vi "FGV_DOCK_controls_state.vi"(7 "options":T1, 8 "error_in":errorcluster, 11 "input":variant) -> (0 "error_out":errorcluster, 3 "output":variant)   [LabVIEW 2019]
uses:
  FGV_DOCK_controls_state.ctl
  FGV_DOCK_controls_state_refnums.ctl
  FGV_DOCK_controls_state_variables.ctl
  _misc/AULocalize/SubVIs/Get Localized Phrase Compact Interface 0D.vi
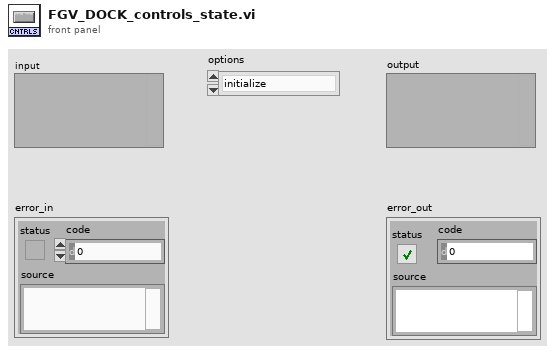
[diagram p1: front panel]
types:
  T1 = typedef "FGV_DOCK_controls_state.ctl" = enum16{"initialize", "login_event", "translation_event", "batch_event", "reload_event", "gear_event", "gear_saved_event", "gear_in_another_batch_event", "gear_in_current_batch_event", "NOK_ref_gear_event", "NOK_station_gear_event", "get_gear_loaded_status"}
  T2 = typedef "FGV_DOCK_controls_state_variables.ctl" = cluster{"access_level":i32, "batch_active?":bool, "gear_loaded?":bool}
  T3 = typedef "FGV_DOCK_controls_state_refnums.ctl" = cluster{"REFERENCE_selector":refnum<vi>, "BATCH_SIZE_selector":refnum<vi>, "DOCK_start_finish_batch":refnum<vi>, "gear_OK":refnum<vi>, "gear_NOK":refnum<vi>, "reload_part_number":refnum<vi>, "reload_batch_size":refnum<vi>, "menu_bar":refnum<k9>}
  T4 = enum8{"Enabled", "Disabled", "Disabled and Grayed Out"}
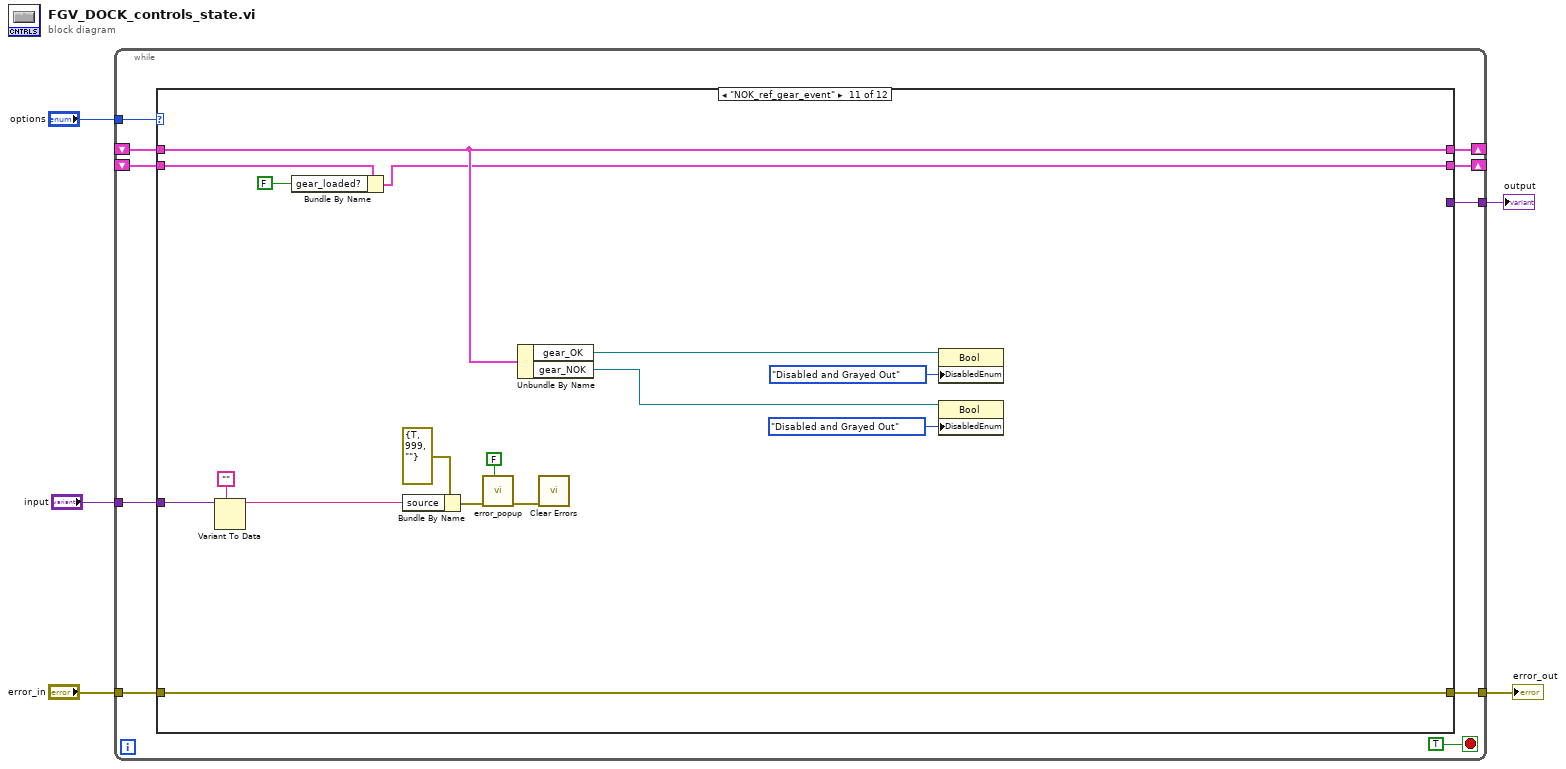
[diagram p0: block diagram]
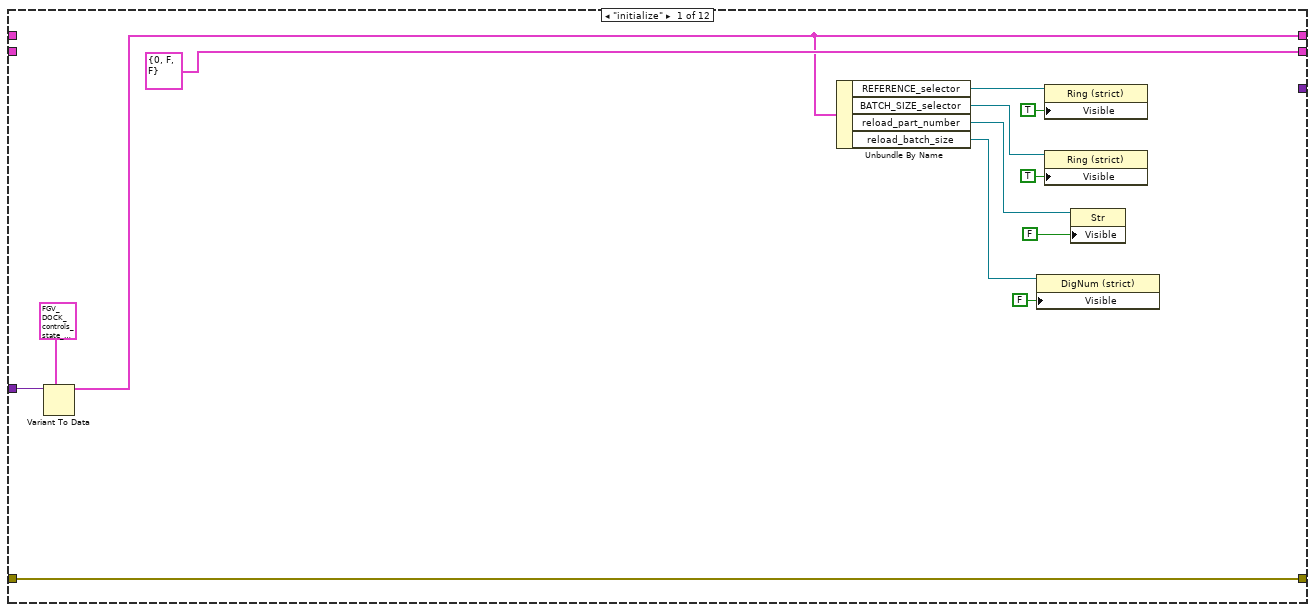
[diagram p2: hidden frame]
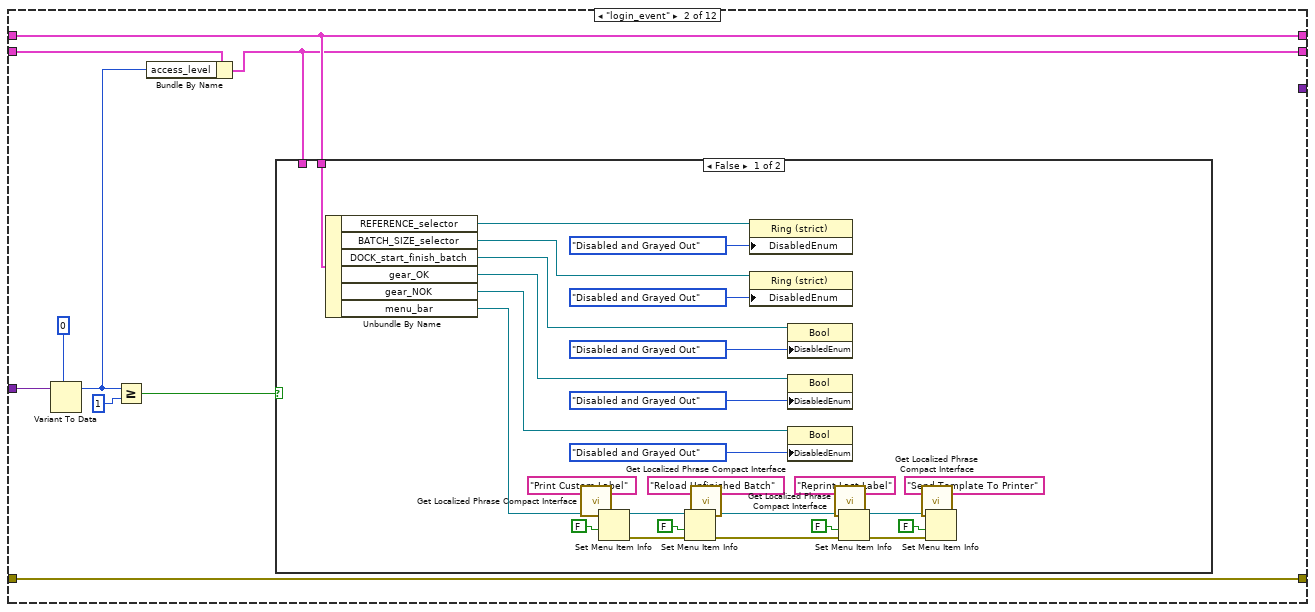
[diagram p3: hidden frame]
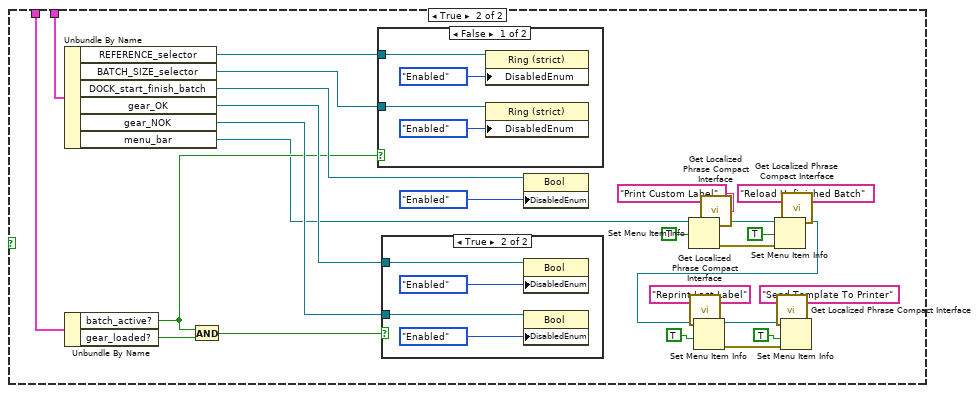
[diagram p4: hidden frame]
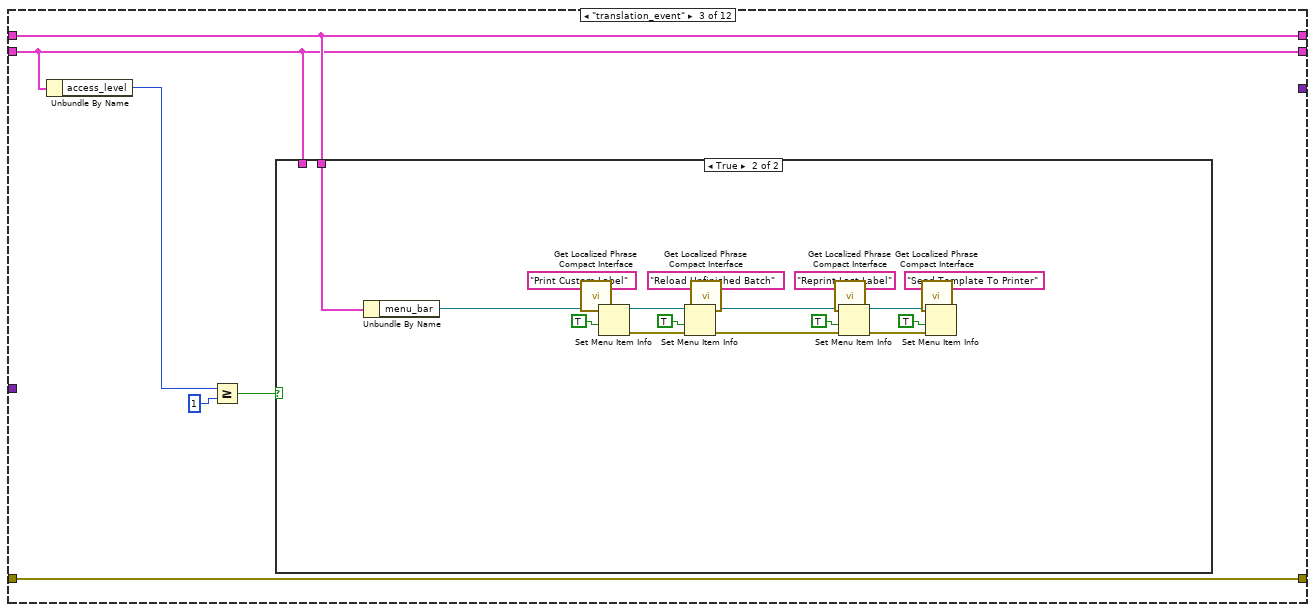
[diagram p7: hidden frame]
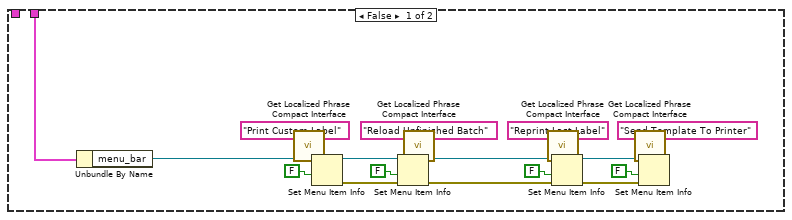
[diagram p8: hidden frame]
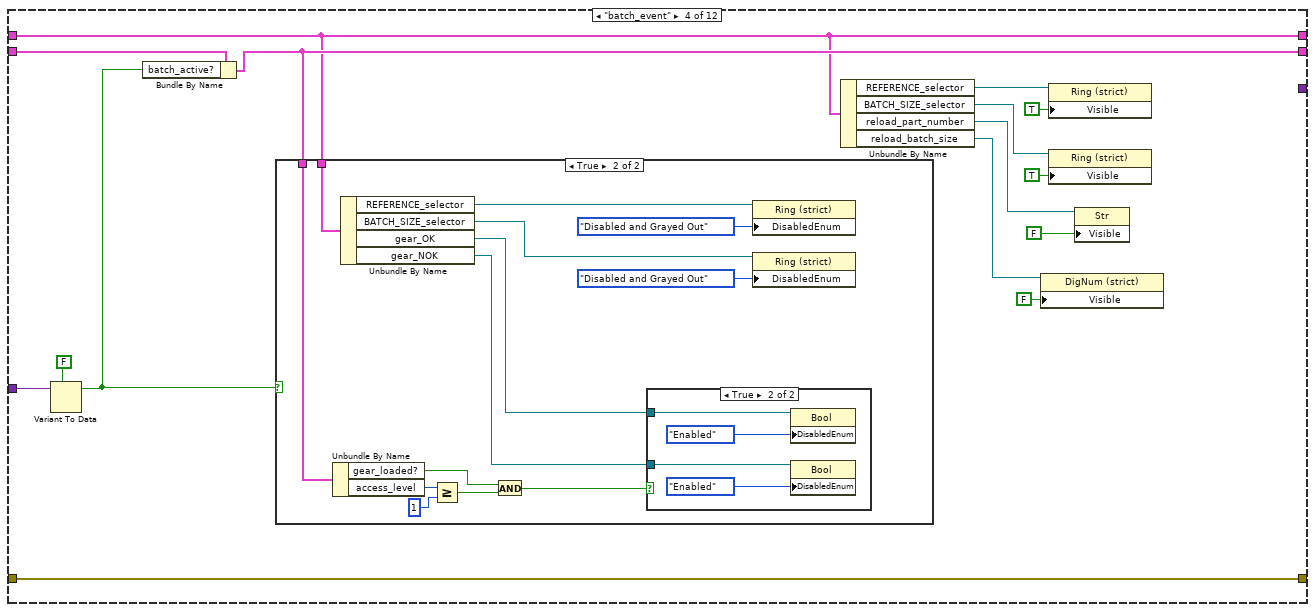
[diagram p9: hidden frame]
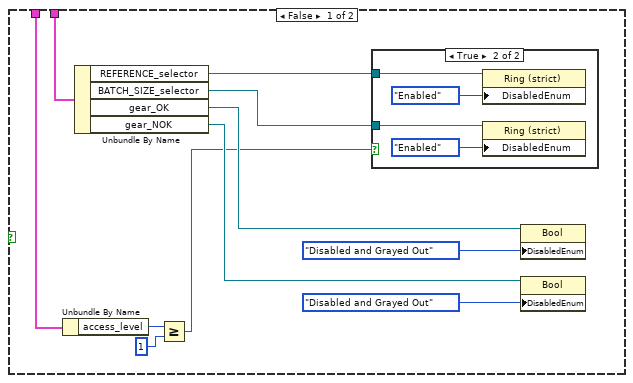
[diagram p10: hidden frame]
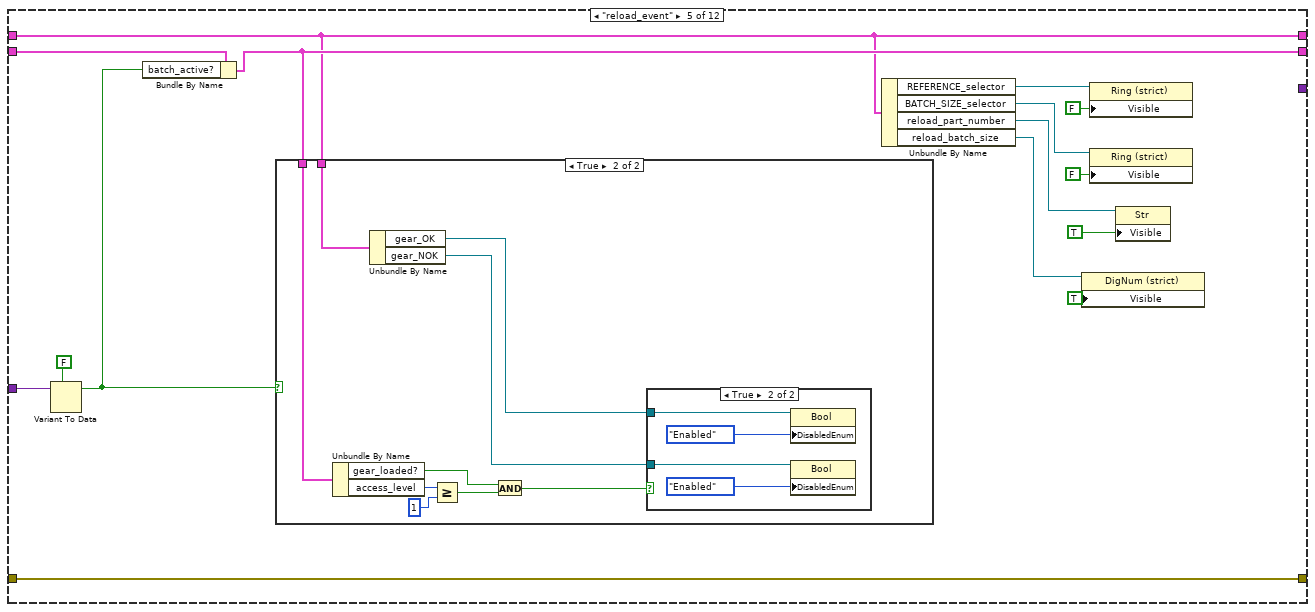
[diagram p13: hidden frame]
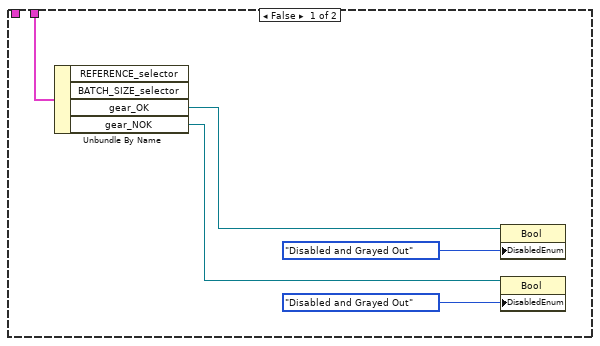
[diagram p14: hidden frame]
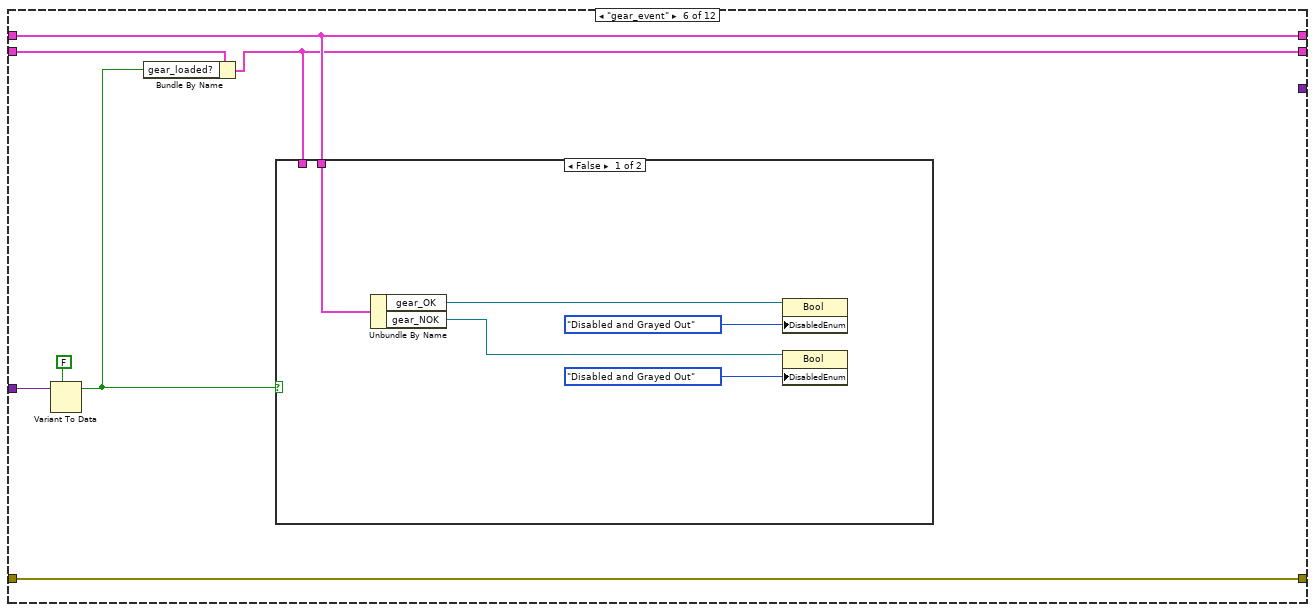
[diagram p16: hidden frame]
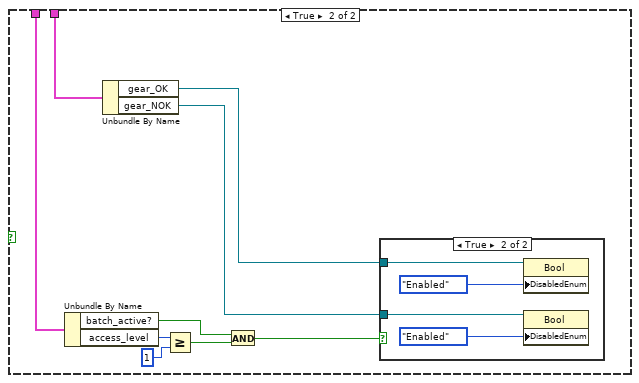
[diagram p17: hidden frame]
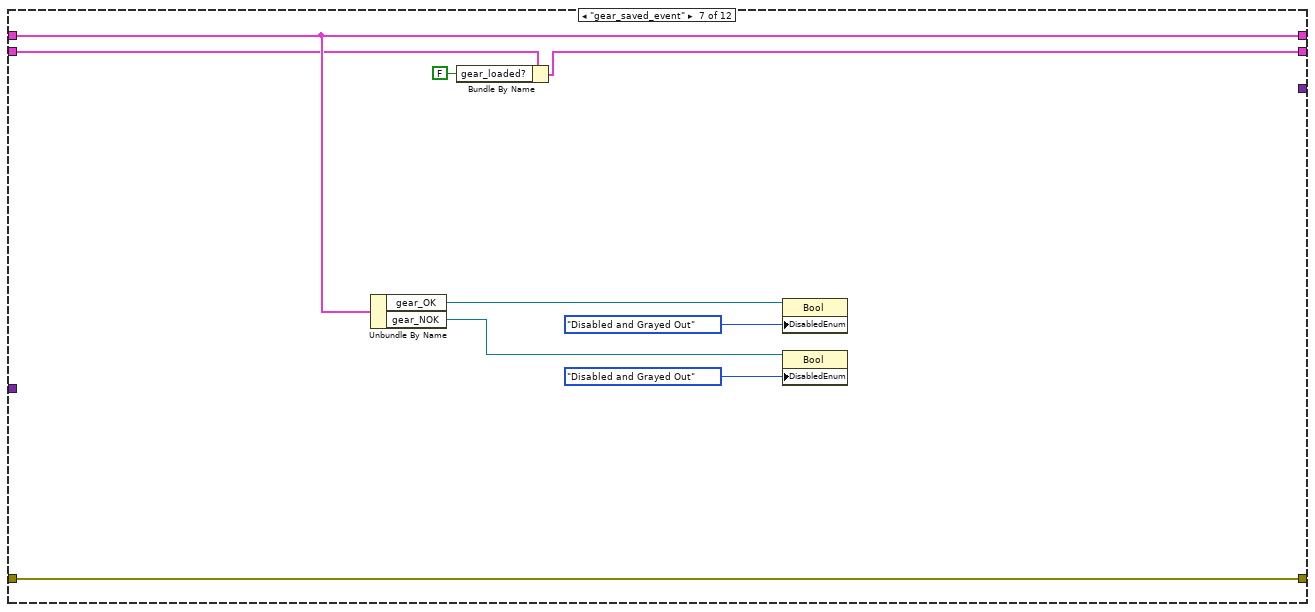
[diagram p19: hidden frame]
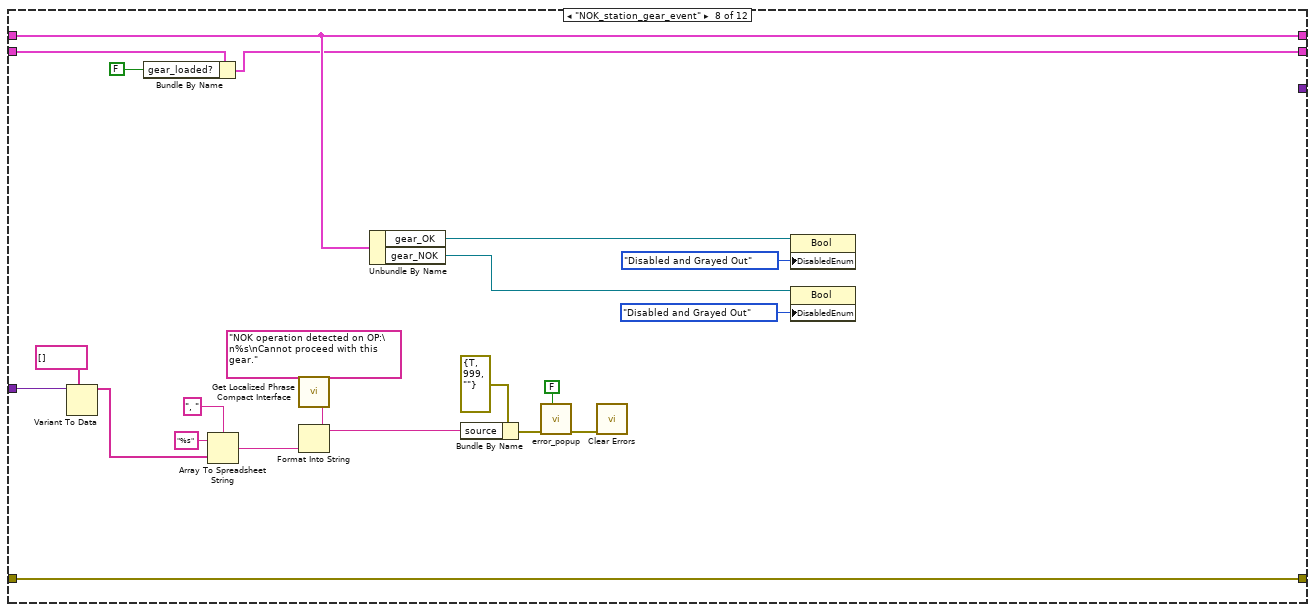
[diagram p20: hidden frame]
diagram:
  n1 = while {
    tunnel: "options" -> [w14]
    tunnel: [w13] -> w5
    tunnel: "error_in" -> [w12]
    tunnel: "input" -> [w11]
    shift-right: [w10] -> _
    shift-left: _ -> [w9]
    shift-right: [w8] -> _
    shift-left: _ -> [w7]
    tunnel: [w6] -> w1
    stop <- TRUE stop-if-true
    n2 = case shown="\"NOK_ref_gear_event\"" w14 {
      tunnel: [w28 w37 w110 w165 w212 w237 w264 w286 w298 w328 w344 w349] -> w13
      tunnel: w12 -> [w28 w37 w110 w165 w212 w237 w264 w286 w298 w328 w344 w349]
      tunnel: w11 -> [w27 w36 _ w164 w211 w236 _ w276 w293 _ w334 _]
      tunnel: [w16 w30 w107 w157 w198 w234 w263 w284 w297 w326 w342 w348] -> w10
      tunnel: w9 -> [_ w30 w107 w157 w198 w234 w263 w284 w297 w326 w342 w348]
      tunnel: [T2 {"access_level"=0, "batch_active?"=FALSE, "gear_loaded?"=FALSE} ("controls_state_variables") w29 w106 w162 w209 w233 w257 w283 w287 w325 w341 w347] -> w8
      tunnel: w7 -> [_ w32 w106 w163 w210 w235 w258 w285 w288 w327 w343 w347]
      tunnel: [_ _ _ _ _ _ _ _ _ _ _ w345] -> w6
      frame "initialize" {
        n3 = Variant To Data(type=T3 {"REFERENCE_selector"=refnum, "BATCH_SIZE_selector"=refnum, "DOCK_start_finish_batch"=refnum, "gear_OK"=refnum, "gear_NOK"=refnum, "reload_part_number"=refnum, "reload_batch_size"=refnum, "menu_bar"=refnum} ("control_refnums"), Variant=w27) -> (data=w16:T3)  [unwired: 1 in, 1 out]
        n4 = Unbundle By Name(w16) -> ("REFERENCE_selector"=w22:refnum<vi>, "BATCH_SIZE_selector"=w21:refnum<vi>, "reload_part_number"=w18:refnum<vi>, "reload_batch_size"=w17:refnum<vi>)
        n5 = property class="DigNum (strict)"(reference=w17, "Visible"=FALSE) -> ()  [unwired: 1 in, 2 out]
        n6 = property class="Ring (strict)"(reference=w22, "Visible"=TRUE) -> ()  [unwired: 1 in, 2 out]
        n7 = property class="Ring (strict)"(reference=w21, "Visible"=TRUE) -> ()  [unwired: 1 in, 2 out]
        n8 = property class="Str"(reference=w18, "Visible"=FALSE) -> ()  [unwired: 1 in, 2 out]
      }
      frame "login_event" {
        n9 = Variant To Data(type=0 ("y"), Variant=w36) -> (data=w31:i32)  [unwired: 1 in, 1 out]
        n10 = Greater Or Equal?(x=w31, y=1) -> (x >= y?=w33:bool)
        n11 = Bundle By Name(cluster=w32, "access_level"=w31) -> (w29:T2)
        n12 = case shown="False" w33 {
          tunnel: w30 -> [w66 w96]
          tunnel: w29 -> [_ w90]
          frame False {
            n13 = Unbundle By Name(w66) -> ("REFERENCE_selector"=w61:refnum<vi>, "BATCH_SIZE_selector"=w60:refnum<vi>, "DOCK_start_finish_batch"=w59:refnum<vi>, "gear_OK"=w58:refnum<vi>, "gear_NOK"=w57:refnum<vi>, "menu_bar"=w50:refnum<k9>)
            n14 = call-poly "Get Localized Phrase Compact Interface.vi"("Key"="Print Custom Label" ("item tag")) -> ("Translated Phrase"=w41:string)
            n15 = Set Menu Item Info(7:w41, 9:FALSE ("enabled"), 11:w50) -> (0:w52:errorcluster, 3:w51:refnum<k9>)  [unwired: 4 in]
            n16 = call-poly "Get Localized Phrase Compact Interface.vi"("Key"="Reload Unfinished Batch" ("item tag")) -> ("Translated Phrase"=w40:string)
            n17 = Set Menu Item Info(7:w40, 8:w52, 9:FALSE ("enabled"), 11:w51) -> (0:w45:errorcluster, 3:w44:refnum<k9>)  [unwired: 3 in]
            n18 = property class="Ring (strict)"(reference=w61, "DisabledEnum"=T4."Disabled and Grayed Out" ("Disabled")) -> ()  [unwired: 1 in, 2 out]
            n19 = property class="Ring (strict)"(reference=w60, "DisabledEnum"=T4."Disabled and Grayed Out" ("Disabled")) -> ()  [unwired: 1 in, 2 out]
            n20 = property class="Bool"(reference=w59, "DisabledEnum"=T4."Disabled and Grayed Out" ("Disabled")) -> ()  [unwired: 1 in, 2 out]
            n21 = property class="Bool"(reference=w58, "DisabledEnum"=T4."Disabled and Grayed Out" ("Disabled")) -> ()  [unwired: 1 in, 2 out]
            n22 = property class="Bool"(reference=w57, "DisabledEnum"=T4."Disabled and Grayed Out" ("Disabled")) -> ()  [unwired: 1 in, 2 out]
            n23 = call-poly "Get Localized Phrase Compact Interface.vi"("Key"="Reprint Last Label") -> ("Translated Phrase"=w39:string)
            n24 = Set Menu Item Info(7:w39, 8:w45, 9:FALSE ("enabled"), 11:w44) -> (0:w48:errorcluster, 3:w49:refnum<k9>)  [unwired: 3 in]
            n25 = call-poly "Get Localized Phrase Compact Interface.vi"("Key"="Send Template To Printer") -> ("Translated Phrase"=w38:string)
            n26 = Set Menu Item Info(7:w38, 8:w48, 9:FALSE ("enabled"), 11:w49) -> ()  [unwired: 3 in, 2 out]
          }
          frame True {
            n27 = Unbundle By Name(w96) -> ("REFERENCE_selector"=w95:refnum<vi>, "BATCH_SIZE_selector"=w94:refnum<vi>, "DOCK_start_finish_batch"=w93:refnum<vi>, "gear_OK"=w92:refnum<vi>, "gear_NOK"=w91:refnum<vi>, "menu_bar"=w79:refnum<k9>)
            n28 = Unbundle By Name(w90) -> ("batch_active?"=w88:bool, "gear_loaded?"=w87:bool)
            n29 = And(x=w88, y=w87) -> (x .and. y?=w86:bool)
            n30 = case shown="False" w88 {
              tunnel: w95 -> [w98 _]
              tunnel: w94 -> [w97 _]
              frame False {
                n31 = property class="Ring (strict)"(reference=w98, "DisabledEnum"=T4."Enabled" ("Disabled")) -> ()  [unwired: 1 in, 2 out]
                n32 = property class="Ring (strict)"(reference=w97, "DisabledEnum"=T4."Enabled" ("Disabled")) -> ()  [unwired: 1 in, 2 out]
              }
              frame True {
              }
            }
            n33 = case shown="True" w86 {
              tunnel: w92 -> [_ w102]
              tunnel: w91 -> [_ w101]
              frame False {
              }
              frame True {
                n34 = property class="Bool"(reference=w102, "DisabledEnum"=T4."Enabled" ("Disabled")) -> ()  [unwired: 1 in, 2 out]
                n35 = property class="Bool"(reference=w101, "DisabledEnum"=T4."Enabled" ("Disabled")) -> ()  [unwired: 1 in, 2 out]
              }
            }
            n36 = property class="Bool"(reference=w93, "DisabledEnum"=T4."Enabled" ("Disabled")) -> ()  [unwired: 1 in, 2 out]
            n37 = call-poly "Get Localized Phrase Compact Interface.vi"("Key"="Reprint Last Label") -> ("Translated Phrase"=w68:string)
            n38 = call-poly "Get Localized Phrase Compact Interface.vi"("Key"="Print Custom Label" ("item tag")) -> ("Translated Phrase"=w71:string)
            n39 = Set Menu Item Info(7:w71, 9:TRUE ("enabled"), 11:w79) -> (0:w85:errorcluster, 3:w84:refnum<k9>)  [unwired: 4 in]
            n40 = call-poly "Get Localized Phrase Compact Interface.vi"("Key"="Send Template To Printer") -> ("Translated Phrase"=w69:string)
            n41 = call-poly "Get Localized Phrase Compact Interface.vi"("Key"="Reload Unfinished Batch" ("item tag")) -> ("Translated Phrase"=w70:string)
            n42 = Set Menu Item Info(7:w70, 8:w85, 9:TRUE ("enabled"), 11:w84) -> (3:w72:refnum<k9>)  [unwired: 3 in, 1 out]
            n43 = Set Menu Item Info(7:w68, 9:TRUE ("enabled"), 11:w72) -> (0:w77:errorcluster, 3:w78:refnum<k9>)  [unwired: 4 in]
            n44 = Set Menu Item Info(7:w69, 8:w77, 9:TRUE ("enabled"), 11:w78) -> ()  [unwired: 3 in, 2 out]
          }
        }
      }
      frame "translation_event" {
        n45 = Unbundle By Name(w106) -> ("access_level"=w105:i32)
        n46 = Greater Or Equal?(x=w105, y=1) -> (x >= y?=w108:bool)
        n47 = case shown="True" w108 {
          tunnel: w107 -> [w130 w150]
          tunnel: w106 -> [_ _]
          frame False {
            n48 = Unbundle By Name(w130) -> ("menu_bar"=w123:refnum<k9>)
            n49 = call-poly "Get Localized Phrase Compact Interface.vi"("Key"="Print Custom Label" ("item tag")) -> ("Translated Phrase"=w114:string)
            n50 = Set Menu Item Info(7:w114, 9:FALSE ("enabled"), 11:w123) -> (0:w125:errorcluster, 3:w124:refnum<k9>)  [unwired: 4 in]
            n51 = call-poly "Get Localized Phrase Compact Interface.vi"("Key"="Reload Unfinished Batch" ("item tag")) -> ("Translated Phrase"=w113:string)
            n52 = Set Menu Item Info(7:w113, 8:w125, 9:FALSE ("enabled"), 11:w124) -> (0:w118:errorcluster, 3:w117:refnum<k9>)  [unwired: 3 in]
            n53 = call-poly "Get Localized Phrase Compact Interface.vi"("Key"="Reprint Last Label") -> ("Translated Phrase"=w112:string)
            n54 = Set Menu Item Info(7:w112, 8:w118, 9:FALSE ("enabled"), 11:w117) -> (0:w121:errorcluster, 3:w122:refnum<k9>)  [unwired: 3 in]
            n55 = call-poly "Get Localized Phrase Compact Interface.vi"("Key"="Send Template To Printer") -> ("Translated Phrase"=w111:string)
            n56 = Set Menu Item Info(7:w111, 8:w121, 9:FALSE ("enabled"), 11:w122) -> ()  [unwired: 3 in, 2 out]
          }
          frame True {
            n57 = Unbundle By Name(w150) -> ("menu_bar"=w143:refnum<k9>)
            n58 = call-poly "Get Localized Phrase Compact Interface.vi"("Key"="Print Custom Label" ("item tag")) -> ("Translated Phrase"=w134:string)
            n59 = Set Menu Item Info(7:w134, 9:TRUE ("enabled"), 11:w143) -> (0:w145:errorcluster, 3:w144:refnum<k9>)  [unwired: 4 in]
            n60 = call-poly "Get Localized Phrase Compact Interface.vi"("Key"="Reload Unfinished Batch" ("item tag")) -> ("Translated Phrase"=w133:string)
            n61 = Set Menu Item Info(7:w133, 8:w145, 9:TRUE ("enabled"), 11:w144) -> (0:w138:errorcluster, 3:w137:refnum<k9>)  [unwired: 3 in]
            n62 = call-poly "Get Localized Phrase Compact Interface.vi"("Key"="Reprint Last Label") -> ("Translated Phrase"=w132:string)
            n63 = Set Menu Item Info(7:w132, 8:w138, 9:TRUE ("enabled"), 11:w137) -> (0:w141:errorcluster, 3:w142:refnum<k9>)  [unwired: 3 in]
            n64 = call-poly "Get Localized Phrase Compact Interface.vi"("Key"="Send Template To Printer") -> ("Translated Phrase"=w131:string)
            n65 = Set Menu Item Info(7:w131, 8:w141, 9:TRUE ("enabled"), 11:w142) -> ()  [unwired: 3 in, 2 out]
          }
        }
      }
      frame "batch_event" {
        n66 = Variant To Data(type=FALSE, Variant=w164) -> (data=w160:bool)  [unwired: 1 in, 1 out]
        n67 = Bundle By Name(cluster=w163, "batch_active?"=w160) -> (w162:T2)
        n68 = case shown="True" w160 {
          tunnel: w157 -> [w176 w193]
          tunnel: w162 -> [w167 w188]
          frame False {
            n69 = Unbundle By Name(w167) -> ("access_level"=w168:i32)
            n70 = Unbundle By Name(w176) -> ("REFERENCE_selector"=w173:refnum<vi>, "BATCH_SIZE_selector"=w172:refnum<vi>, "gear_OK"=w171:refnum<vi>, "gear_NOK"=w170:refnum<vi>)
            n71 = Greater Or Equal?(x=w168, y=1) -> (x >= y?=w166:bool)
            n72 = case shown="True" w166 {
              tunnel: w173 -> [_ w178]
              tunnel: w172 -> [_ w177]
              frame False {
              }
              frame True {
                n73 = property class="Ring (strict)"(reference=w178, "DisabledEnum"=T4."Enabled" ("Disabled")) -> ()  [unwired: 1 in, 2 out]
                n74 = property class="Ring (strict)"(reference=w177, "DisabledEnum"=T4."Enabled" ("Disabled")) -> ()  [unwired: 1 in, 2 out]
              }
            }
            n75 = property class="Bool"(reference=w171, "DisabledEnum"=T4."Disabled and Grayed Out" ("Disabled")) -> ()  [unwired: 1 in, 2 out]
            n76 = property class="Bool"(reference=w170, "DisabledEnum"=T4."Disabled and Grayed Out" ("Disabled")) -> ()  [unwired: 1 in, 2 out]
          }
          frame True {
            n77 = Unbundle By Name(w188) -> ("gear_loaded?"=w182:bool, "access_level"=w184:i32)
            n78 = Unbundle By Name(w193) -> ("REFERENCE_selector"=w192:refnum<vi>, "BATCH_SIZE_selector"=w191:refnum<vi>, "gear_OK"=w190:refnum<vi>, "gear_NOK"=w189:refnum<vi>)
            n79 = Greater Or Equal?(x=w184, y=1) -> (x >= y?=w183:bool)
            n80 = And(x=w182, y=w183) -> (x .and. y?=w181:bool)
            n81 = case shown="True" w181 {
              tunnel: w190 -> [_ w197]
              tunnel: w189 -> [_ w196]
              frame False {
              }
              frame True {
                n82 = property class="Bool"(reference=w197, "DisabledEnum"=T4."Enabled" ("Disabled")) -> ()  [unwired: 1 in, 2 out]
                n83 = property class="Bool"(reference=w196, "DisabledEnum"=T4."Enabled" ("Disabled")) -> ()  [unwired: 1 in, 2 out]
              }
            }
            n84 = property class="Ring (strict)"(reference=w192, "DisabledEnum"=T4."Disabled and Grayed Out" ("Disabled")) -> ()  [unwired: 1 in, 2 out]
            n85 = property class="Ring (strict)"(reference=w191, "DisabledEnum"=T4."Disabled and Grayed Out" ("Disabled")) -> ()  [unwired: 1 in, 2 out]
          }
        }
        n86 = Unbundle By Name(w157) -> ("REFERENCE_selector"=w156:refnum<vi>, "BATCH_SIZE_selector"=w155:refnum<vi>, "reload_part_number"=w152:refnum<vi>, "reload_batch_size"=w151:refnum<vi>)
        n87 = property class="DigNum (strict)"(reference=w151, "Visible"=FALSE) -> ()  [unwired: 1 in, 2 out]
        n88 = property class="Ring (strict)"(reference=w156, "Visible"=TRUE) -> ()  [unwired: 1 in, 2 out]
        n89 = property class="Ring (strict)"(reference=w155, "Visible"=TRUE) -> ()  [unwired: 1 in, 2 out]
        n90 = property class="Str"(reference=w152, "Visible"=FALSE) -> ()  [unwired: 1 in, 2 out]
      }
      frame "reload_event" {
        n91 = Variant To Data(type=FALSE, Variant=w211) -> (data=w207:bool)  [unwired: 1 in, 1 out]
        n92 = Bundle By Name(cluster=w210, "batch_active?"=w207) -> (w209:T2)
        n93 = case shown="True" w207 {
          tunnel: w198 -> [w217 w226]
          tunnel: w209 -> [_ w223]
          frame False {
            n94 = Unbundle By Name(w217) -> ("gear_OK"=w214:refnum<vi>, "gear_NOK"=w213:refnum<vi>)  [unwired: 2 out]
            n95 = property class="Bool"(reference=w214, "DisabledEnum"=T4."Disabled and Grayed Out" ("Disabled")) -> ()  [unwired: 1 in, 2 out]
            n96 = property class="Bool"(reference=w213, "DisabledEnum"=T4."Disabled and Grayed Out" ("Disabled")) -> ()  [unwired: 1 in, 2 out]
          }
          frame True {
            n97 = Unbundle By Name(w223) -> ("gear_loaded?"=w219:bool, "access_level"=w221:i32)
            n98 = Unbundle By Name(w226) -> ("gear_OK"=w225:refnum<vi>, "gear_NOK"=w224:refnum<vi>)
            n99 = Greater Or Equal?(x=w221, y=1) -> (x >= y?=w220:bool)
            n100 = And(x=w219, y=w220) -> (x .and. y?=w218:bool)
            n101 = case shown="True" w218 {
              tunnel: w225 -> [_ w230]
              tunnel: w224 -> [_ w229]
              frame False {
              }
              frame True {
                n102 = property class="Bool"(reference=w230, "DisabledEnum"=T4."Enabled" ("Disabled")) -> ()  [unwired: 1 in, 2 out]
                n103 = property class="Bool"(reference=w229, "DisabledEnum"=T4."Enabled" ("Disabled")) -> ()  [unwired: 1 in, 2 out]
              }
            }
          }
        }
        n104 = Unbundle By Name(w198) -> ("REFERENCE_selector"=w204:refnum<vi>, "BATCH_SIZE_selector"=w203:refnum<vi>, "reload_part_number"=w200:refnum<vi>, "reload_batch_size"=w199:refnum<vi>)
        n105 = property class="DigNum (strict)"(reference=w199, "Visible"=TRUE) -> ()  [unwired: 1 in, 2 out]
        n106 = property class="Ring (strict)"(reference=w204, "Visible"=FALSE) -> ()  [unwired: 1 in, 2 out]
        n107 = property class="Ring (strict)"(reference=w203, "Visible"=FALSE) -> ()  [unwired: 1 in, 2 out]
        n108 = property class="Str"(reference=w200, "Visible"=TRUE) -> ()  [unwired: 1 in, 2 out]
      }
      frame "gear_event" {
        n109 = Variant To Data(type=FALSE, Variant=w236) -> (data=w231:bool)  [unwired: 1 in, 1 out]
        n110 = Bundle By Name(cluster=w235, "gear_loaded?"=w231) -> (w233:T2)
        n111 = case shown="False" w231 {
          tunnel: w234 -> [w242 w251]
          tunnel: w233 -> [_ w248]
          frame False {
            n112 = Unbundle By Name(w242) -> ("gear_OK"=w239:refnum<vi>, "gear_NOK"=w238:refnum<vi>)
            n113 = property class="Bool"(reference=w239, "DisabledEnum"=T4."Disabled and Grayed Out" ("Disabled")) -> ()  [unwired: 1 in, 2 out]
            n114 = property class="Bool"(reference=w238, "DisabledEnum"=T4."Disabled and Grayed Out" ("Disabled")) -> ()  [unwired: 1 in, 2 out]
          }
          frame True {
            n115 = Unbundle By Name(w248) -> ("batch_active?"=w244:bool, "access_level"=w246:i32)
            n116 = Unbundle By Name(w251) -> ("gear_OK"=w250:refnum<vi>, "gear_NOK"=w249:refnum<vi>)
            n117 = Greater Or Equal?(x=w246, y=1) -> (x >= y?=w245:bool)
            n118 = And(x=w244, y=w245) -> (x .and. y?=w243:bool)
            n119 = case shown="True" w243 {
              tunnel: w250 -> [_ w255]
              tunnel: w249 -> [_ w254]
              frame False {
              }
              frame True {
                n120 = property class="Bool"(reference=w255, "DisabledEnum"=T4."Enabled" ("Disabled")) -> ()  [unwired: 1 in, 2 out]
                n121 = property class="Bool"(reference=w254, "DisabledEnum"=T4."Enabled" ("Disabled")) -> ()  [unwired: 1 in, 2 out]
              }
            }
          }
        }
      }
      frame "gear_saved_event" {
        n122 = Unbundle By Name(w263) -> ("gear_OK"=w260:refnum<vi>, "gear_NOK"=w259:refnum<vi>)
        n123 = Bundle By Name(cluster=w258, "gear_loaded?"=FALSE) -> (w257:T2)
        n124 = property class="Bool"(reference=w260, "DisabledEnum"=T4."Disabled and Grayed Out" ("Disabled")) -> ()  [unwired: 1 in, 2 out]
        n125 = property class="Bool"(reference=w259, "DisabledEnum"=T4."Disabled and Grayed Out" ("Disabled")) -> ()  [unwired: 1 in, 2 out]
      }
      frame "NOK_station_gear_event" {
        n126 = Variant To Data(type=string[] [], Variant=w276) -> (data=w270:string[])  [unwired: 1 in, 1 out]
        n127 = Bundle By Name(cluster=w285, "gear_loaded?"=FALSE) -> (w283:T2)
        n128 = Array To Spreadsheet String(delimiter (Tab)=", ", array=w270, 3:"%s" ("format string")) -> (spreadsheet string=w269:string)
        n129 = call-poly "Get Localized Phrase Compact Interface.vi"("Key"="NOK operation detected on OP:\n%s\nCannot proceed with this gear." ("format string")) -> ("Translated Phrase"=w265:string)
        n130 = Format Into String(format string=w265, w269) -> (resulting string=w268:string)  [unwired: 2 in, 1 out]
        n131 = Unbundle By Name(w284) -> ("gear_OK"=w281:refnum<vi>, "gear_NOK"=w280:refnum<vi>)
        n132 = Bundle By Name(cluster=errorcluster {"status"=TRUE, "code"=999, "source"=""} ("error_in"), "source"=w268) -> (w273:errorcluster)
        n133 = call "error_popup.vi"("EXIT App If Error? (F)"=FALSE, "error_in"=w273) -> ("error_out"=w266:errorcluster)  [unwired: 9 in]
        n134 = call <vilib>:"Clear Errors.vi"("error in (no error)"=w266) -> ()  [unwired: 5 in, 2 out]
        n135 = property class="Bool"(reference=w281, "DisabledEnum"=T4."Disabled and Grayed Out" ("Disabled")) -> ()  [unwired: 1 in, 2 out]
        n136 = property class="Bool"(reference=w280, "DisabledEnum"=T4."Disabled and Grayed Out" ("Disabled")) -> ()  [unwired: 1 in, 2 out]
      }
      frame "gear_in_another_batch_event" {
        n137 = Variant To Data(type=0 ("current_access_level"), Variant=w293) -> (data=w291:i32)  [unwired: 1 in, 1 out]
        n138 = Greater Or Equal?(x=w291, y=2) -> (x >= y?=w289:bool)
        n139 = case shown="True" w289 {
          tunnel: [T4."Disabled and Grayed Out" ("Disabled") T4."Enabled" ("Disabled")] -> w294
          tunnel: w288 -> [w301 w309]
          tunnel: [w299 w308] -> w287
          frame False {
            n140 = Bundle By Name(cluster=errorcluster {"status"=TRUE, "code"=999, "source"=""} ("error_in"), "source"="Selected gear is already assigned to another batch.\nYour access level is too low to reassign it.\nTo reassign this gear log in with higher access level." ("format string")) -> (w305:errorcluster)
            n141 = call "error_popup.vi"("EXIT App If Error? (F)"=FALSE, "error_in"=w305) -> ("error_out"=w304:errorcluster)  [unwired: 9 in]
            n142 = call <vilib>:"Clear Errors.vi"("error in (no error)"=w304) -> ()  [unwired: 5 in, 2 out]
            n143 = Bundle By Name(cluster=w301, "gear_loaded?"=FALSE) -> (w299:T2)
          }
          frame True {
            n144 = call "message_popup.vi"("Warning(T)/Info(F)"=TRUE, "Message"="This gear is already assigned to another batch.\nYou access level allows you to reassign it to current batch in the next window, but make sure this is what you want before doing so.", "Title"="Warning", "Button Label"="OK") -> ()  [unwired: 7 in, 1 out]
            n145 = Bundle By Name(cluster=w309, "gear_loaded?"=TRUE) -> (w308:T2)
          }
        }
        n146 = Unbundle By Name(w297) -> ("gear_OK"=w296:refnum<vi>, "gear_NOK"=w295:refnum<vi>)
        n147 = property class="Bool"(reference=w296, "DisabledEnum"=w294) -> ()  [unwired: 1 in, 2 out]
        n148 = property class="Bool"(reference=w295, "DisabledEnum"=w294) -> ()  [unwired: 1 in, 2 out]
      }
      frame "gear_in_current_batch_event" {
        w321 = T4."Disabled and Grayed Out" ("Disabled")
        n149 = Bundle By Name(cluster=w327, "gear_loaded?"=FALSE) -> (w325:T2)
        n150 = Unbundle By Name(w326) -> ("gear_OK"=w323:refnum<vi>, "gear_NOK"=w322:refnum<vi>)
        n151 = Bundle By Name(cluster=errorcluster {"status"=TRUE, "code"=999, "source"=""} ("error_in"), "source"="Selected gear is already assigned to current batch." ("format string")) -> (w318:errorcluster)
        n152 = call "error_popup.vi"("EXIT App If Error? (F)"=FALSE, "error_in"=w318) -> ("error_out"=w317:errorcluster)  [unwired: 9 in]
        n153 = property class="Bool"(reference=w323, "DisabledEnum"=w321) -> ()  [unwired: 1 in, 2 out]
        n154 = property class="Bool"(reference=w322, "DisabledEnum"=w321) -> ()  [unwired: 1 in, 2 out]
        n155 = call <vilib>:"Clear Errors.vi"("error in (no error)"=w317) -> ()  [unwired: 5 in, 2 out]
      }
      frame "NOK_ref_gear_event" {
        n156 = Variant To Data(type="", Variant=w334) -> (data=w329:string)  [unwired: 1 in, 1 out]
        n157 = Bundle By Name(cluster=w343, "gear_loaded?"=FALSE) -> (w341:T2)
        n158 = Bundle By Name(cluster=errorcluster {"status"=TRUE, "code"=999, "source"=""} ("error_in"), "source"=w329) -> (w332:errorcluster)
        n159 = call "error_popup.vi"("EXIT App If Error? (F)"=FALSE, "error_in"=w332) -> ("error_out"=w331:errorcluster)  [unwired: 9 in]
        n160 = Unbundle By Name(w342) -> ("gear_OK"=w339:refnum<vi>, "gear_NOK"=w338:refnum<vi>)
        n161 = call <vilib>:"Clear Errors.vi"("error in (no error)"=w331) -> ()  [unwired: 5 in, 2 out]
        n162 = property class="Bool"(reference=w339, "DisabledEnum"=T4."Disabled and Grayed Out" ("Disabled")) -> ()  [unwired: 1 in, 2 out]
        n163 = property class="Bool"(reference=w338, "DisabledEnum"=T4."Disabled and Grayed Out" ("Disabled")) -> ()  [unwired: 1 in, 2 out]
      }
      frame "get_gear_loaded_status" {
        n164 = Unbundle By Name(w347) -> ("gear_loaded?"=w346:bool)
        n165 = To Variant(anything=w346) -> (Variant=w345:variant)
      }
    }
  }
  "error_out" <- w5
  "output" <- w1
